vi "5800PRSet.vi"() -> ()   [LabVIEW 2022 SP3]
doc: "This application VI allows the user to set the desired parameters in the \n5800 / 5900 P / R. just select thevalues that you want to set the instrument to from the 5800 / 5900 user interface and click on the send to 5800 button."
uses:
  Motion Controllers/-MotionRoutines/MotionGlobals.vi
panel:
  in  "Output Att":dbl=5.0 min=0.0 max=15.9 step=0.1 format="%.1g"
  in  "Gain":u16(ring) items=["20.0 dB", "40.0 dB", "60.0 dB"]
  in  "Input Att":u16(ring)=1 items=["0.0 dB", "10.0 dB", "20.0 dB", "30.0 dB", "40.0 dB", "50.0 dB"]
  in  "Lowpass Filter":u16(ring)=3 items=["5 MHz", "10 MHz", "20 MHz", "35 MHz"]
  in  "Highpass Filter":u16(ring) items=["1 KHz", "100 KHz", "300 KHz", "1000 KHz"]
  in  "Damping Value":u16(ring)=3 items=["15 ohms", "17 ohms", "21 ohms", "25 ohms", "36 ohms", "50 ohms", "100 ohms", "500 ohms"]
  in  "Energy Level":u16(ring)=1 items=["12.5 uJ", "25.0 uJ", "50.0 uJ", "100.0 uJ"]
  in  "PRF":u16(ring)=10 items=["External Remote", "External BNC", "0.080 KHz", "0.100 KHz", "0.125 KHz", "0.160 KHz", "0.200 KHz", "0.250 KHz", "0.400 KHz", "0.500 KHz", "1.000 KHz", "1.250 KHz", "2.000 KHz", "2.500 KHz", "4.000 KHz", "5.000 KHz", "10.000 KHz", "OFF"]
  in  "Operation Mode":u16(ring) items=["Pulse-Echo", "Through", "External Pulser"]
  in  "ExitSendCmd":bool
  # "MODEL 5800"
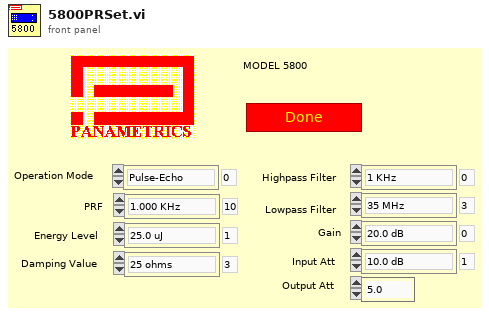
[diagram p1: front panel]
types:
  T1 = typedef "location.ctl" = enum16{"Automatic", "WCM Main", "Hawaii", "Columbia MM3000", "Columbia  NI System", "NYU", "RRI 2", "UHI Allen", "CUMC RT", "Chiba", "Stony Brook", "WCM Microscopy", "WCM Aeoretch", "WCM Optics Lab", "WCM Main 2Axis", "WCM Rotation", "WCM SAM SMAC", "SERI GP"}
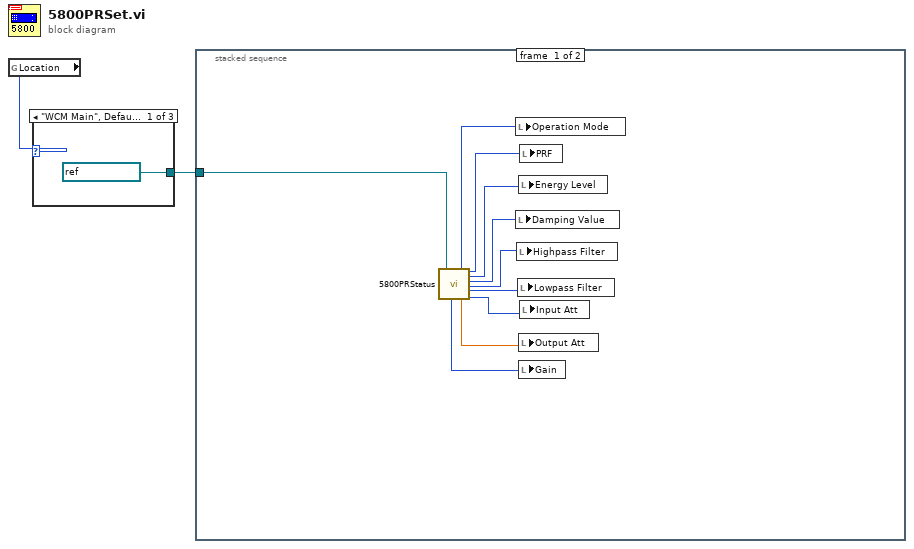
[diagram p0: block diagram]
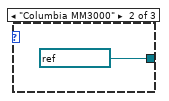
[diagram p2: hidden frame]
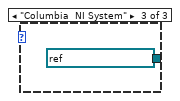
[diagram p3: hidden frame]
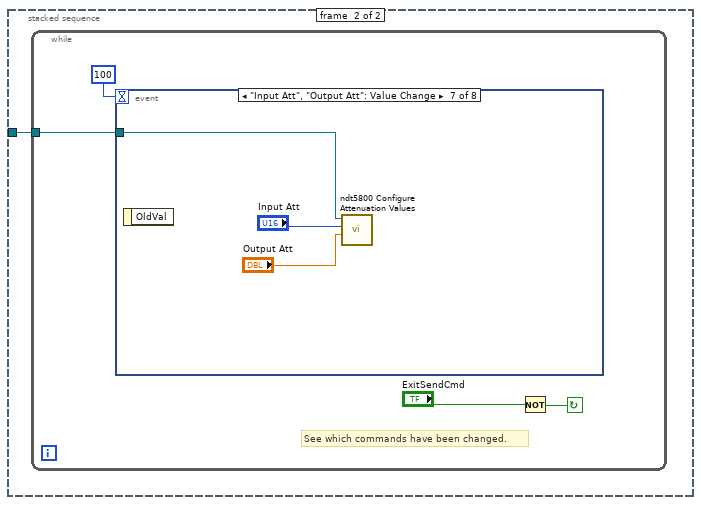
[diagram p4: hidden frame]
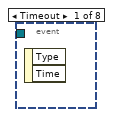
[diagram p5: hidden frame]
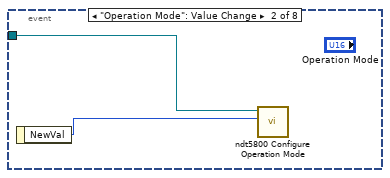
[diagram p6: hidden frame]
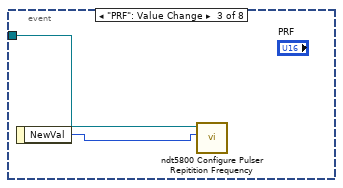
[diagram p7: hidden frame]
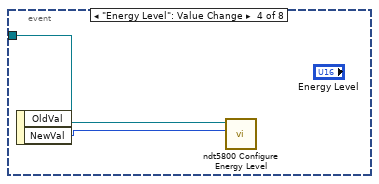
[diagram p8: hidden frame]
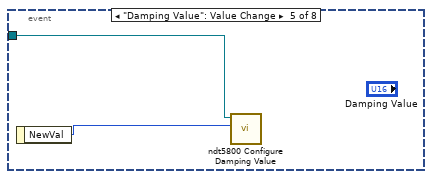
[diagram p9: hidden frame]
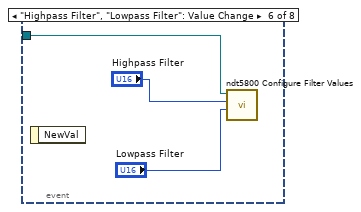
[diagram p10: hidden frame]
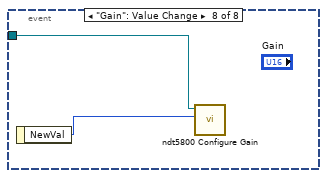
[diagram p11: hidden frame]
diagram:
  n1 = global read "MotionGlobals.vi" "Location"() -> (w1:T1)
  n2 = case shown="\"WCM Main\", Default" w1 {
    tunnel: [refnum<visa-resource-name> "GPIB::1" ("VISA resource name") refnum<visa-resource-name> "GPIB0::9" ("VISA resource name") refnum<visa-resource-name> "GPIB0::9::INSTR" ("VISA resource name")] -> w2
    frame "WCM Main", Default {
    }
    frame "Columbia MM3000" {
    }
    frame "Columbia  NI System" {
    }
  }
  n3 = stacked-sequence {
    tunnel: w2 -> [w15 w16]
    frame #0 {
      n4 = call "5800PRStatus.vi"("VISA resource name"=w15) -> ("Gain"=w6:u16, "Operation Mode"=w14:u16, "Output Attenuation"=w7:dbl, "Pulser Repitition Frequency"=w13:u16, "Energy Level"=w12:u16, "Damping Value"=w11:u16, "Highpass Filter Frequency"=w10:u16, "Lowpass Filter Frequency"=w9:u16, "Input Attenuation"=w8:u16)  [unwired: 8 in, 2 out]
      n5 = local write "Operation Mode"(w14) -> ()
      n6 = local write "Damping Value"(w11) -> ()
      n7 = local write "Highpass Filter"(w10) -> ()
      n8 = local write "Lowpass Filter"(w9) -> ()
      n9 = local write "Energy Level"(w12) -> ()
      n10 = local write "Output Att"(w7) -> ()
      n11 = local write "Gain"(w6) -> ()
      n12 = local write "PRF"(w13) -> ()
      n13 = local write "Input Att"(w8) -> ()
    }
    frame #1 {
      n14 = while {
        tunnel: w16 -> [w17]
        stop <- w20 continue-if-true
        # "See which commands have been changed."
        n15 = event shown="[6] \"Input Att\", \"Output Att\": Value Change" {
          selector: _ -> [_ _ _ _ _ _ _ _]
          dyn-events: _ -> [_ _ _ _ _ _ _ _]
          timeout: 100 -> [_ _ _ _ _ _ _ _]
          tunnel: w17 -> [_ w22 w23 w25 w27 w31 w34 w36]
          event Timeout {
            n16 = event-data() -> ()  [unwired: 3 out]
          }
          event "Operation Mode": Value Change {
            n17 = event-data() -> ("NewVal"=w21:u16)  [unwired: 1 out]
            n18 = call <instrlib>:"ndt5800 Configure Operation Mode.vi"("Operation Mode (Pulse-Echo)"=w21, "VISA resource name"=w22) -> ()  [unwired: 8 in, 2 out]
          }
          event "PRF": Value Change {
            n19 = event-data() -> ("NewVal"=w24:u16)  [unwired: 1 out]
            n20 = call <instrlib>:"ndt5800 Configure Pulser Repitition Frequency.vi"("Pulser Repitition Frequency (1.000 KHz)"=w24, "VISA resource name"=w23) -> ()  [unwired: 8 in, 2 out]
          }
          event "Energy Level": Value Change {
            n21 = event-data() -> ("NewVal"=w26:u16)  [unwired: 2 out]
            n22 = call <instrlib>:"ndt5800 Configure Energy Level.vi"("Energy Level (25.0 uJ)"=w26, "VISA resource name"=w25) -> ()  [unwired: 8 in, 2 out]
          }
          event "Damping Value": Value Change {
            n23 = event-data() -> ("NewVal"=w28:u16)  [unwired: 1 out]
            n24 = call <instrlib>:"ndt5800 Configure Damping Value.vi"("Damping Value (25 ohms)"=w28, "VISA resource name"=w27) -> ()  [unwired: 8 in, 2 out]
          }
          event "Highpass Filter", "Lowpass Filter": Value Change {
            n25 = event-data() -> ()  [unwired: 2 out]
            n26 = call <instrlib>:"ndt5800 Configure Filter Values.vi"("Lowpass Filter Frequency (35 MHz)"="Lowpass Filter", "Highpass Filter Frequency (1 KHz)"="Highpass Filter", "VISA resource name"=w31) -> ()  [unwired: 7 in, 2 out]
          }
          event "Input Att", "Output Att": Value Change {
            n27 = event-data() -> ()  [unwired: 2 out]
            n28 = call <instrlib>:"ndt5800 Configure Attenuation Values.vi"("Output Attenuation (5.0 dB)"="Output Att", "Input Attenuation (10.0 dB)"="Input Att", "VISA resource name"=w34) -> ()  [unwired: 7 in, 2 out]
          }
          event "Gain": Value Change {
            n29 = event-data() -> ("NewVal"=w35:u16)  [unwired: 1 out]
            n30 = call <instrlib>:"ndt5800 Configure Gain.vi"("Gain (20.0 dB)"=w35, "VISA resource name"=w36) -> ()  [unwired: 8 in, 2 out]
          }
        }
        n31 = Not(x="ExitSendCmd") -> (.not. x?=w20:bool)
      }
    }
  }
